vi "leerEETTdesdeBD.vi"(8 "error in (no error)":errorcluster, 11 "Sonometro in":refnum<class "Sonometro.lvclass">) -> (0 "error out":errorcluster, 3 "Sonometro out":refnum<class "Sonometro.lvclass">)   [LabVIEW 2019, in "Sonometro.lvclass"]
uses:
  Sonometro.lvclass
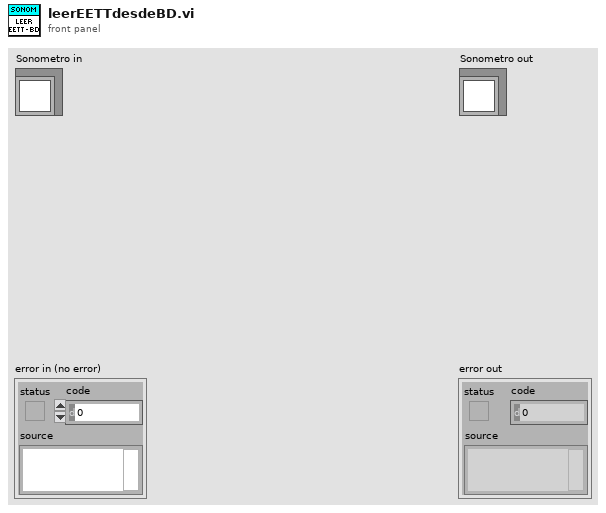
[diagram p1: front panel]
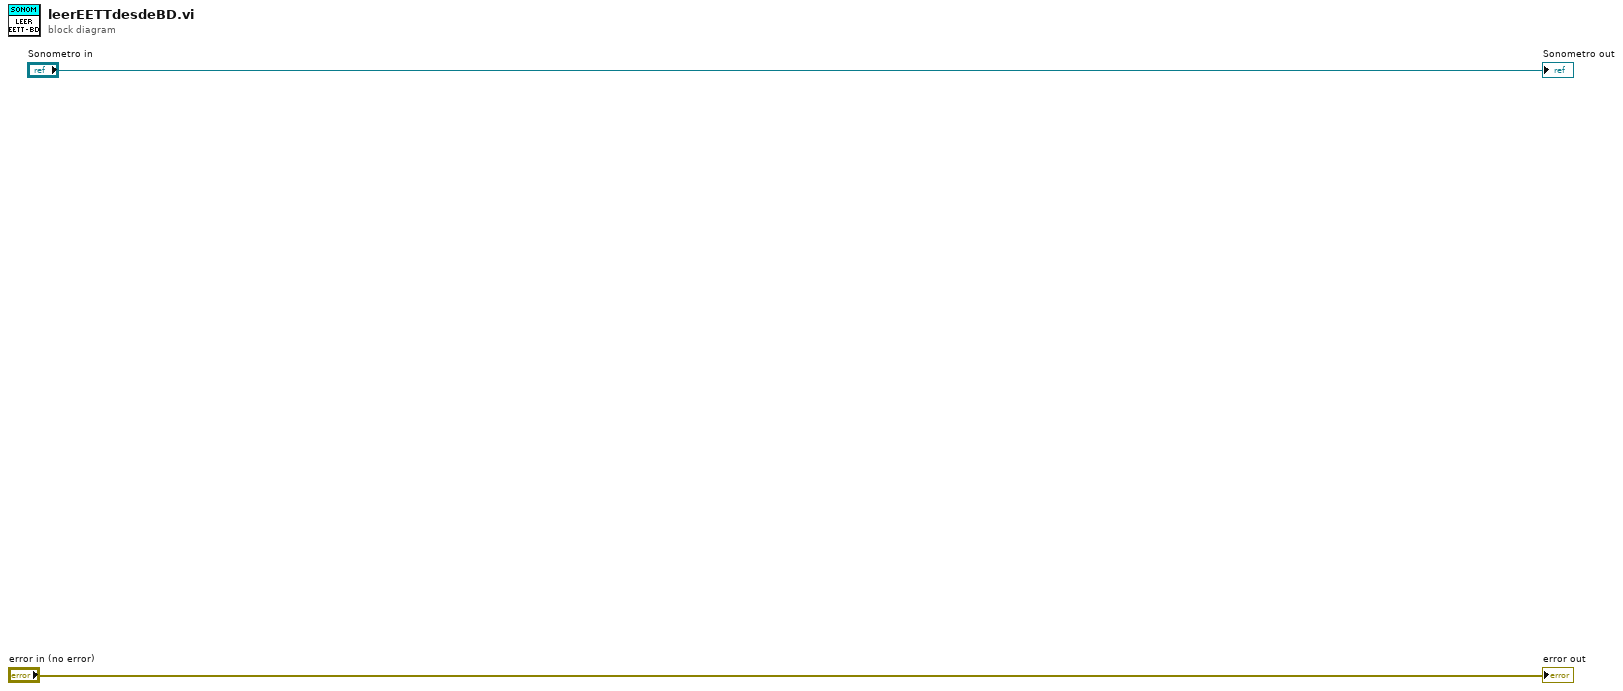
[diagram p0: block diagram]
diagram:
  "error out" <- "error in (no error)"
  "Sonometro out" <- "Sonometro in"
